vi "Constructor.vi"(10 "Capacity":u32) -> (3 "TypedCircularBuffer out":refnum<class "RotateCircularBuffer.lvclass">)   [LabVIEW 2024, in "RotateCircularBuffer.lvclass"]
uses:
  RotateCircularBuffer.lvclass
  RotateCircularBuffer.lvclass/RotateCircularBuffer.ctl
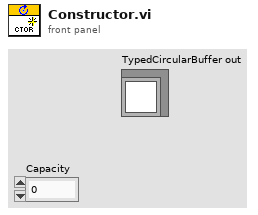
[diagram p1: front panel]
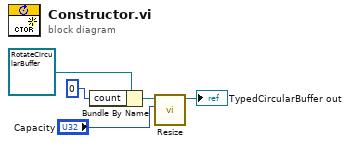
[diagram p0: block diagram]
diagram:
  n1 = Bundle By Name(cluster=refnum<class "RotateCircularBuffer.lvclass"> refnum ("TypedCircularBuffer.lvclass"), "count"=u32 0 ("size")) -> (w4:refnum<class "RotateCircularBuffer.lvclass">)
  n2 = call "Resize.vi"("Capacity"="Capacity", "TypedCircularBuffer in"=w4) -> ("TypedCircularBuffer out"=→"TypedCircularBuffer out":refnum<class "RotateCircularBuffer.lvclass">)  [unwired: 9 in]
